vi "Read_Value_Arduino.vi"(3 "error in (no error)":errorcluster, 4 "write buffer":string, 5 "VISA resource name":refnum<visa-resource-name>) -> (0 "error out":errorcluster, 1 "read buffer":string, 2 "VISA resource name out":refnum<visa-resource-name>)   [LabVIEW 2018]
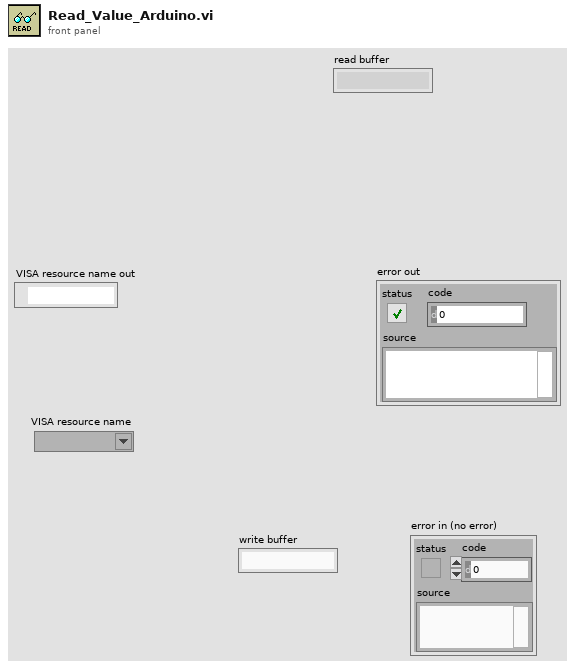
[diagram p1: front panel]
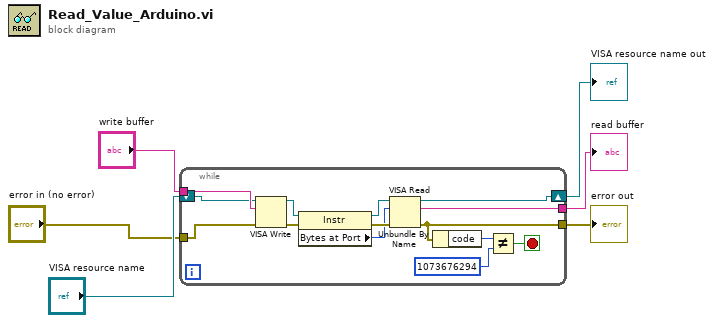
[diagram p0: block diagram]
diagram:
  n1 = while {
    tunnel: "write buffer" -> [w14]
    tunnel: [w11] -> w5
    shift-right: [w10] -> w4
    shift-left: "VISA resource name" -> [w8]
    tunnel: [w9] -> w2
    tunnel: "error in (no error)" -> [w7]
    stop <- w17 stop-if-true
    n2 = VISA Write(VISA resource name=w8, write buffer=w14, error in (no error)=w7) -> (VISA resource name out=w20:refnum<visa-resource-name>, error out=w19:errorcluster)  [unwired: 1 out]
    n3 = property class="Instr"(reference=w20, error in=w19) -> (reference out=w12:refnum<visa-resource-name>, error out=w18:errorcluster, "Bytes at Port"=w13:u32)
    n4 = VISA Read(VISA resource name=w12, byte count=w13, error in (no error)=w18) -> (VISA resource name out=w10:refnum<visa-resource-name>, read buffer=w11:string, error out=w9:errorcluster)  [unwired: 1 out]
    n5 = Unbundle By Name(w9) -> ("code"=w16:i32)
    n6 = Not Equal?(x=w16, y=1073676294) -> (x != y?=w17:bool)
  }
  "error out" <- w2
  "VISA resource name out" <- w4
  "read buffer" <- w5
